vi "mining perform search.vi"(8 "error in (no error)":errorcluster, 9 "sxScenarioId (\"\")":string, 10 "Action (\"Search\")":string="Search", 11 "Connection Refnum":T4) -> (0 "error out":errorcluster, 1 "Matching Results":i32, 2 "Results":T1[](array[typedef]), 3 "Connection Refnum":T4)   [LabVIEW 2011]
uses:
  SI.LIB/ODBC/SQL Controls/Connection Refnum.ctl
  server/database/Scenarios/Scenario Record.ctl
  server/database/Scenarios/Conditions/Condition Record.ctl
  server/database/Scenarios/Conditions/Condition Operators.ctl
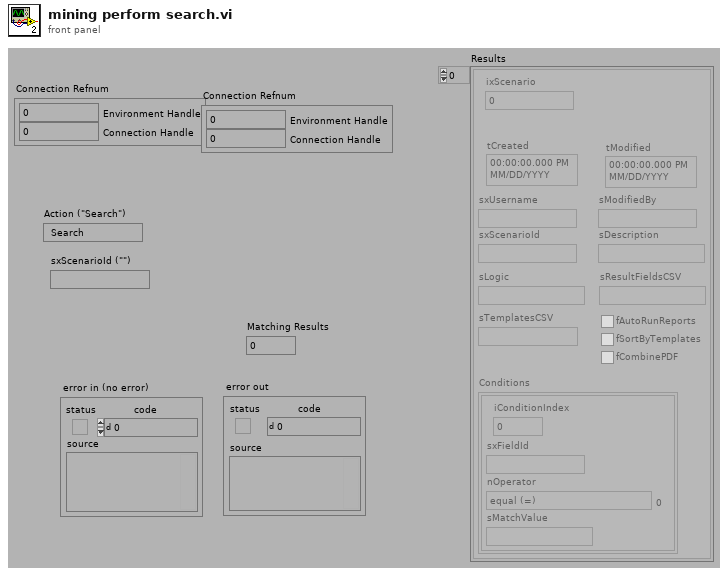
[diagram p1: front panel]
types:
  T1 = typedef "Scenario Record.ctl" = cluster{"ixScenario":i32, "tCreated":timestamp, "tModified":timestamp, "sxUsername":string, "sModifiedBy":string, "sxScenarioId":string, "sDescription":string, "sLogic":string, "sResultFieldsCSV":string, "sTemplatesCSV":string, "fAutoRunReports":bool, "fSortByTemplates":bool, "fCombinePDF":bool, "Conditions":T2[]}
  T2 = typedef "Condition Record.ctl" = cluster{"iConditionIndex":i32, "sxFieldId":string, "nOperator":T3, "sMatchValue":string}
  T3 = typedef "Condition Operators.ctl" = enum16{"equal (=)", "not equal (\\u2260)", "less than (<)", "less than or equal (\\u2264)", "greater than (>)", "greater than or equal (\\u2265)", "contains", "does not contain"}
  T4 = typedef "Connection Refnum.ctl" = cluster{"Environment Handle":i32, "Connection Handle":i32}
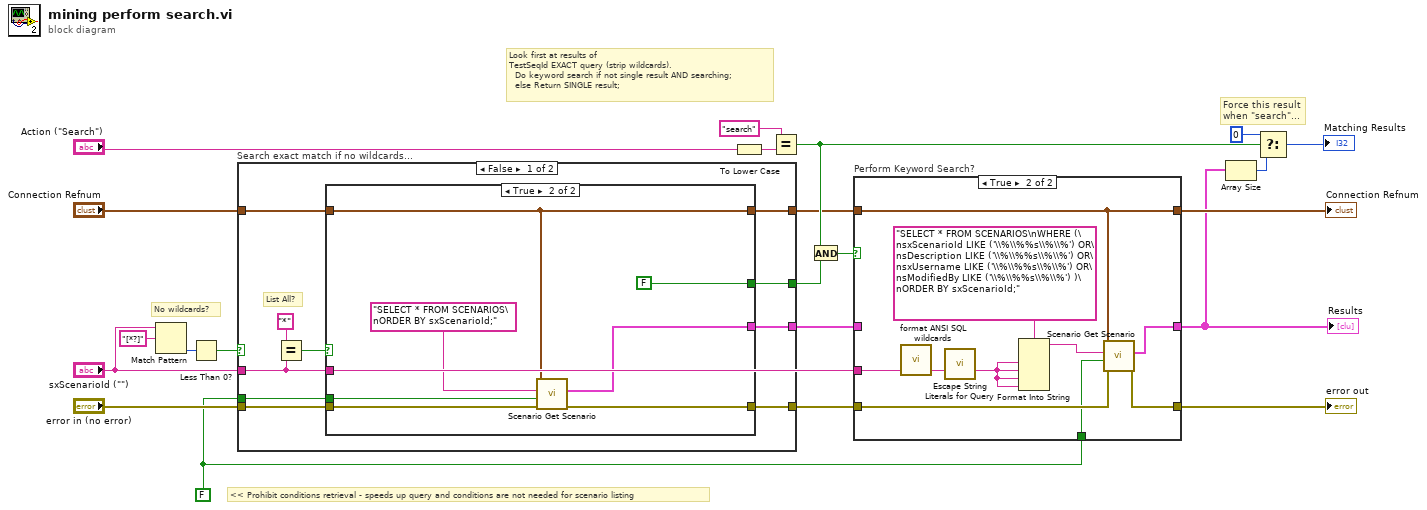
[diagram p0: block diagram]
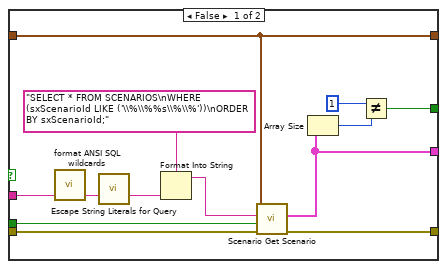
[diagram p2: hidden frame]
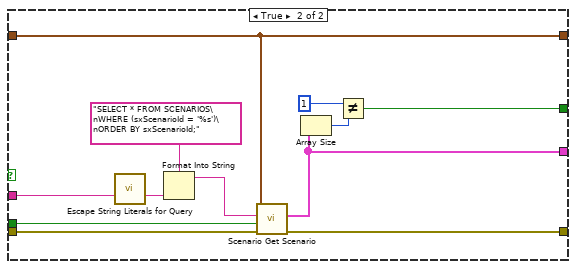
[diagram p3: hidden frame]
diagram:
  w1 = FALSE
  # "<< Prohibit conditions retrieval - speeds up query and conditions are not needed for scenario listing"
  # "No wildcards?"
  # "Force this result\nwhen \"search\"..."
  # "Look first at results of\nTestSeqId EXACT query (strip wildcards).\n  Do keyword search if not single result AND searching;\n  else Return SINGLE result;"
  n1 = Match Pattern(string="sxScenarioId (\"\")", regular expression="[*?]") -> (offset past match=w13:i32)  [unwired: 4 out]
  n2 = Less Than 0?(x=w13) -> (x < 0?=w11:bool)
  n3 = case "Search exact match if no wildcards..." shown="False" w11 {
    tunnel: "error in (no error)" -> [w30 w59]
    tunnel: [w29 w58] -> w8
    tunnel: "Connection Refnum" -> [w28 w56]
    tunnel: [w26 w56] -> w9
    tunnel: [w32 w61] -> w6
    tunnel: [w27 w57] -> w7
    tunnel: "sxScenarioId (\"\")" -> [w25 w60]
    tunnel: w1 -> [w23 w53]
    frame False {
      # "List All?"
      n4 = Equal?(x="*" ("regular expression"), y=w25) -> (x = y?=w31:bool)
      n5 = case shown="True" w31 {
        tunnel: [w40 FALSE] -> w32
        tunnel: w30 -> [w39 w51]
        tunnel: [w38 w50] -> w29
        tunnel: w28 -> [w37 w49]
        tunnel: [w36 w47] -> w27
        tunnel: [w37 w49] -> w26
        tunnel: w25 -> [w41 _]
        tunnel: w23 -> [w33 w46]
        frame False {
          n6 = call "format ANSI SQL wildcards.vi"("String"=w41) -> ("ANSI SQL Wildcard String"=w45:string)  [unwired: 4 out]
          n7 = call "Escape String Literals for Query.vi"("String"=w45) -> ("escaped String"=w44:string)  [unwired: 1 in, 13 out]
          n8 = Format Into String(format string="SELECT * FROM SCENARIOS\nWHERE (sxScenarioId LIKE ('\\%\\%%s\\%\\%'))\nORDER BY sxScenarioId;" ("User Query"), w44) -> (resulting string=w35:string)  [unwired: 2 in, 1 out]
          n9 = call "Scenario Get Scenario.vi"("error in (no error)"=w39, "Retrieve Conditions? (t)"=w33, "Query"=w35, "Connection Refnum"=w37) -> ("error out"=w38:errorcluster, "Scenarios"=w36:T1[])  [unwired: 6 out]
          n10 = Array Size(array=w36) -> (size(s)=w42:i32)
          n11 = Not Equal?(x=1, y=w42) -> (x != y?=w40:bool)
        }
        frame True {
          n12 = call "Scenario Get Scenario.vi"("error in (no error)"=w51, "Retrieve Conditions? (t)"=w46, "Query"="SELECT * FROM SCENARIOS\nORDER BY sxScenarioId;" ("User Query"), "Connection Refnum"=w49) -> ("error out"=w50:errorcluster, "Scenarios"=w47:T1[])  [unwired: 6 out]
        }
      }
    }
    frame True {
      n13 = call "Escape String Literals for Query.vi"("String"=w60) -> ("escaped String"=w64:string)  [unwired: 1 in, 13 out]
      n14 = Format Into String(format string="SELECT * FROM SCENARIOS\nWHERE (sxScenarioId = '%s')\nORDER BY sxScenarioId;" ("User Query"), w64) -> (resulting string=w55:string)  [unwired: 2 in, 1 out]
      n15 = call "Scenario Get Scenario.vi"("error in (no error)"=w59, "Retrieve Conditions? (t)"=w53, "Query"=w55, "Connection Refnum"=w56) -> ("error out"=w58:errorcluster, "Scenarios"=w57:T1[])  [unwired: 6 out]
      n16 = Array Size(array=w57) -> (size(s)=w62:i32)
      n17 = Not Equal?(x=1, y=w62) -> (x != y?=w61:bool)
    }
  }
  n18 = To Lower Case(string="Action (\"Search\")") -> (all lower case string=w4:string)
  n19 = Equal?(x="search", y=w4) -> (x = y?=w18:bool)
  n20 = And(x=w18, y=w6) -> (x .and. y?=w21:bool)
  n21 = case "Perform Keyword Search?" shown="True" w21 {
    tunnel: w9 -> [w66 w75]
    tunnel: w8 -> [w65 w72]
    tunnel: [w66 w75] -> w20
    tunnel: "sxScenarioId (\"\")" -> [_ w76]
    tunnel: w7 -> [w67 _]
    tunnel: [w67 w74] -> w2
    tunnel: [w65 w71] -> w19
    tunnel: w1 -> [_ w69]
    frame False {
    }
    frame True {
      n22 = call "format ANSI SQL wildcards.vi"("String"=w76) -> ("ANSI SQL Wildcard String"=w77:string)  [unwired: 4 out]
      n23 = call "Escape String Literals for Query.vi"("String"=w77) -> ("escaped String"=w68:string)  [unwired: 1 in, 13 out]
      n24 = Format Into String(format string="SELECT * FROM SCENARIOS\nWHERE (\nsxScenarioId LIKE ('\\%\\%%s\\%\\%') OR\nsDescription LIKE ('\\%\\%%s\\%\\%') OR\nsxUsername LIKE ('\\%\\%%s\\%\\%') OR\nsModifiedBy LIKE ('\\%\\%%s\\%\\%') )\nORDER BY sxScenarioId;" ("User Query"), w68, w68, w68, w68) -> (resulting string=w73:string)  [unwired: 2 in, 1 out]
      n25 = call "Scenario Get Scenario.vi"("error in (no error)"=w72, "Retrieve Conditions? (t)"=w69, "Query"=w73, "Connection Refnum"=w75) -> ("error out"=w71:errorcluster, "Scenarios"=w74:T1[])  [unwired: 6 out]
    }
  }
  "error out" <- w19
  "Connection Refnum" <- w20
  "Results" <- w2
  n26 = Array Size(array=w2) -> (size(s)=w17:i32)
  n27 = Select(t=0, s=w18, f=w17) -> (s? t:f=→"Matching Results":i32)
